vi "IsPadConnected.vi"(10 "Input":T1, 11 "Pad Number":i32) -> (3 "Connected?":bool)   [LabVIEW 2012, in "Virtual-PGA.lvlib"]
uses:
  Virtual-PGA.lvlib
  Public/Controls/Input.ctl
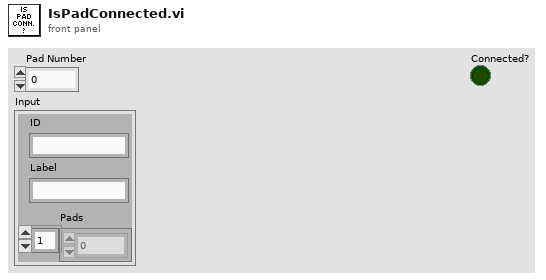
[diagram p1: front panel]
types:
  T1 = typedef "Virtual-PGA.lvlib/Input.ctl" = cluster{"ID":string, "Label":string, "Pads":u32[]}
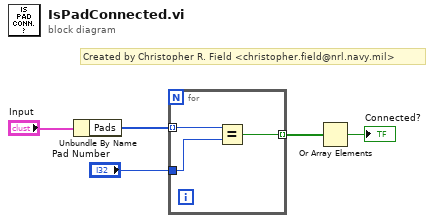
[diagram p0: block diagram]
diagram:
  # "Created by Christopher R. Field <christopher.field@nrl.navy.mil>"
  n1 = Unbundle By Name("Input") -> ("Pads"=w4:u32[])
  n2 = for {
    tunnel: w4 -> [w8] mode=indexing
    tunnel: "Pad Number" -> [w7]
    tunnel: [w6] -> w2 mode=indexing
    n3 = Equal?(x=w8, y=w7) -> (x = y?=w6:bool)
  }
  n4 = Or Array Elements(Boolean array=w2) -> (logical OR=→"Connected?":bool)
